vi "CorrelationTest2.vi"() -> ()   [LabVIEW 2014]
uses:
  <userlib>/Nanonis Prog Interface V5/Nanonis Prog Interface.lvlib
  <vilib>/Analysis/NI_AALPro.lvlib
  <vilib>/Analysis/2dsp.llb/2D Cross Correlation (DBL).vi
panel:
  out "Pixelated 2":picture
  out "Y drift 2":i32
  out "X drift 2":i32
  out "Pixelated":picture
  in  "length":i32
  in  "Boolean 2":bool
  in  "Filter order (2)":i32=2 min=1 max=1000 step=1
  in  "Cutoff frq (0.125)":dbl=0.125
  out "Array 2":dbl[][](array[numeric])
  out "min index(es)":i32[](array[numeric])
  in  "Numeric":i32
  out "shifted":picture
  out "Y drift":i32
  out "X drift":i32
  in  "method":i32 min=0 max=5
  in  "Boolean":bool
  out "Array":dbl[][](array[numeric])
  out "Rxy":dbl[][](array[numeric])
  out "max index(es)":i32[](array[numeric])=[127, 127]
  out "error":i32
  out "norm":picture
  out "no norm":picture
  in  "Read channel 2":i8 min=-1
  in  "algorithm":enum32{"direct", "frequency domain"}(ring)=enum."frequency domain"
  out "Correlation":picture
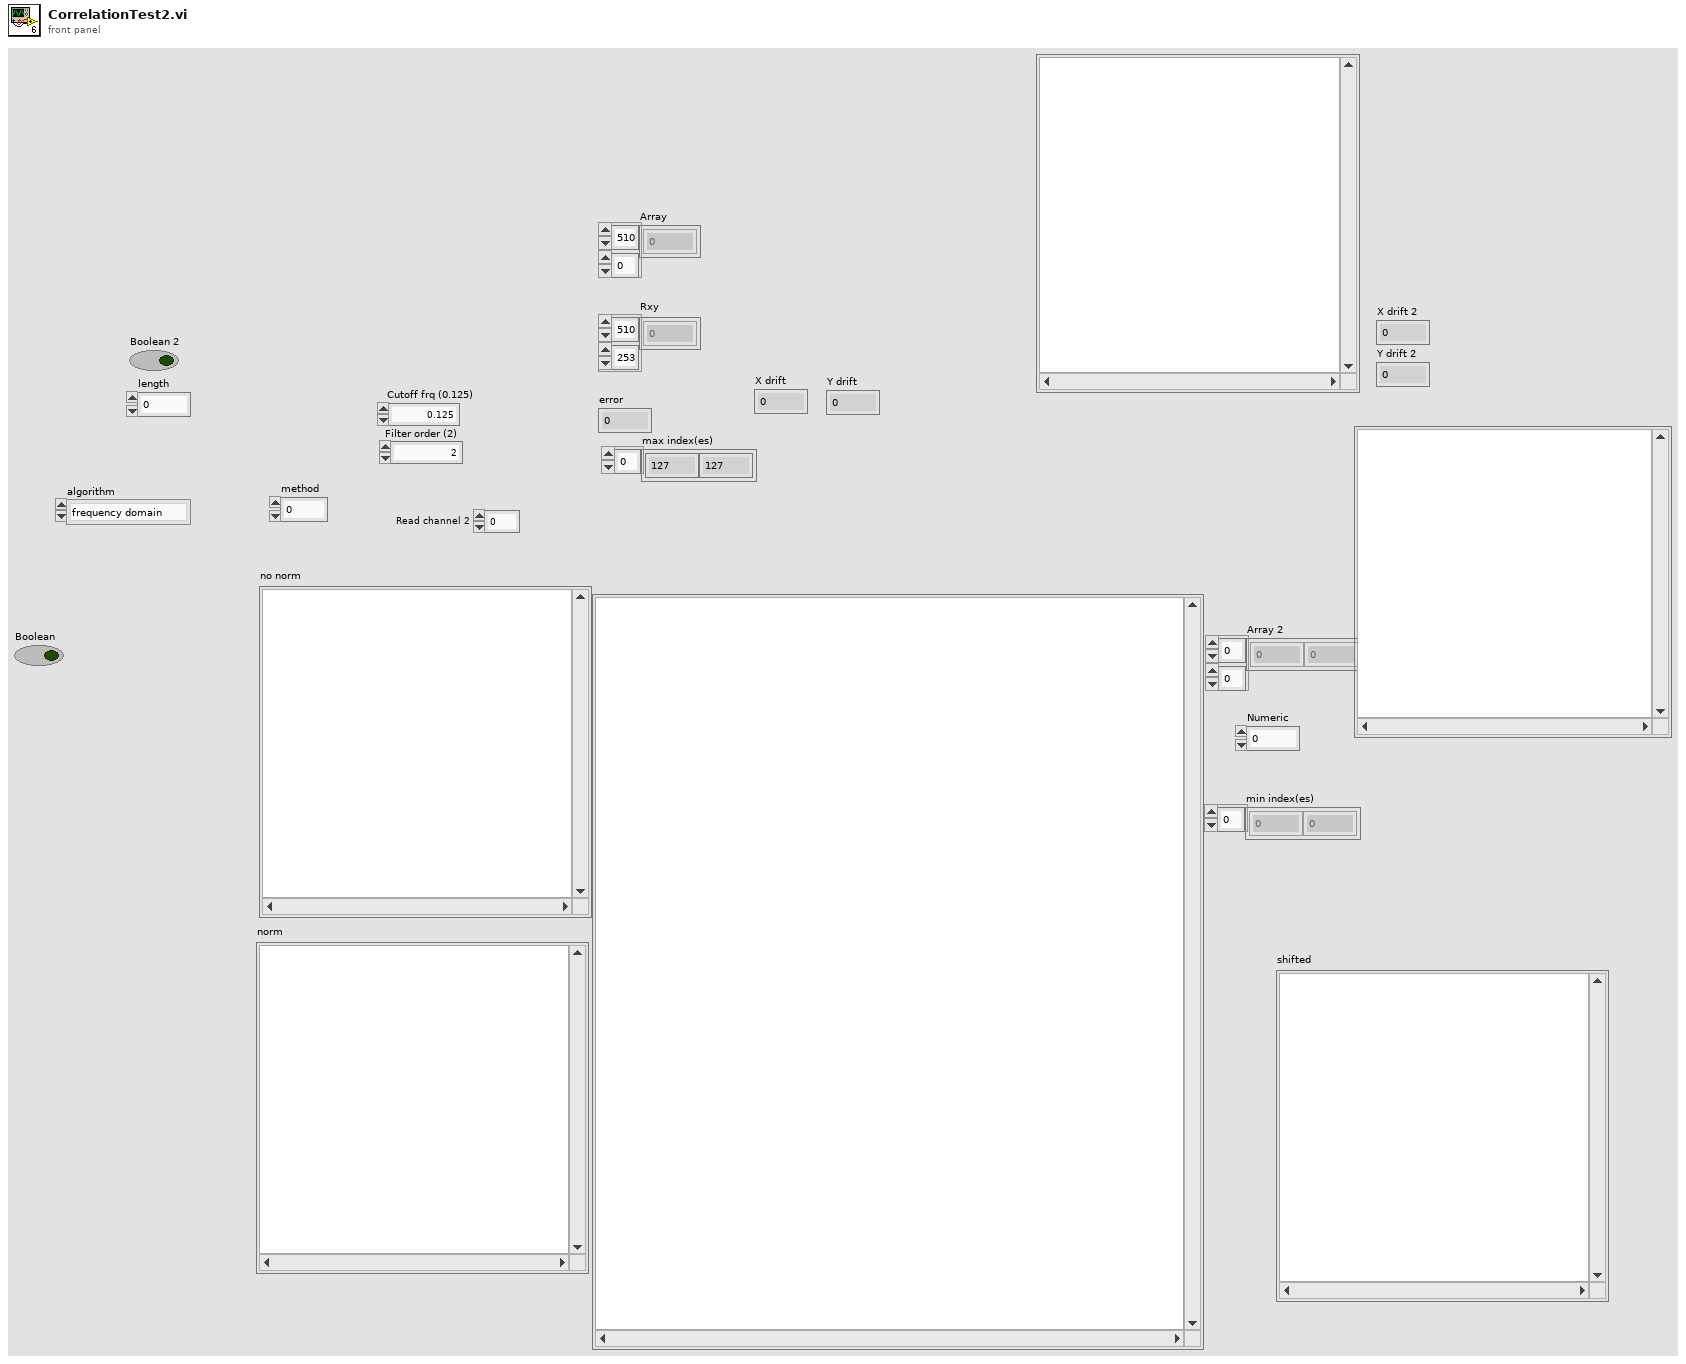
[diagram p1: front panel]
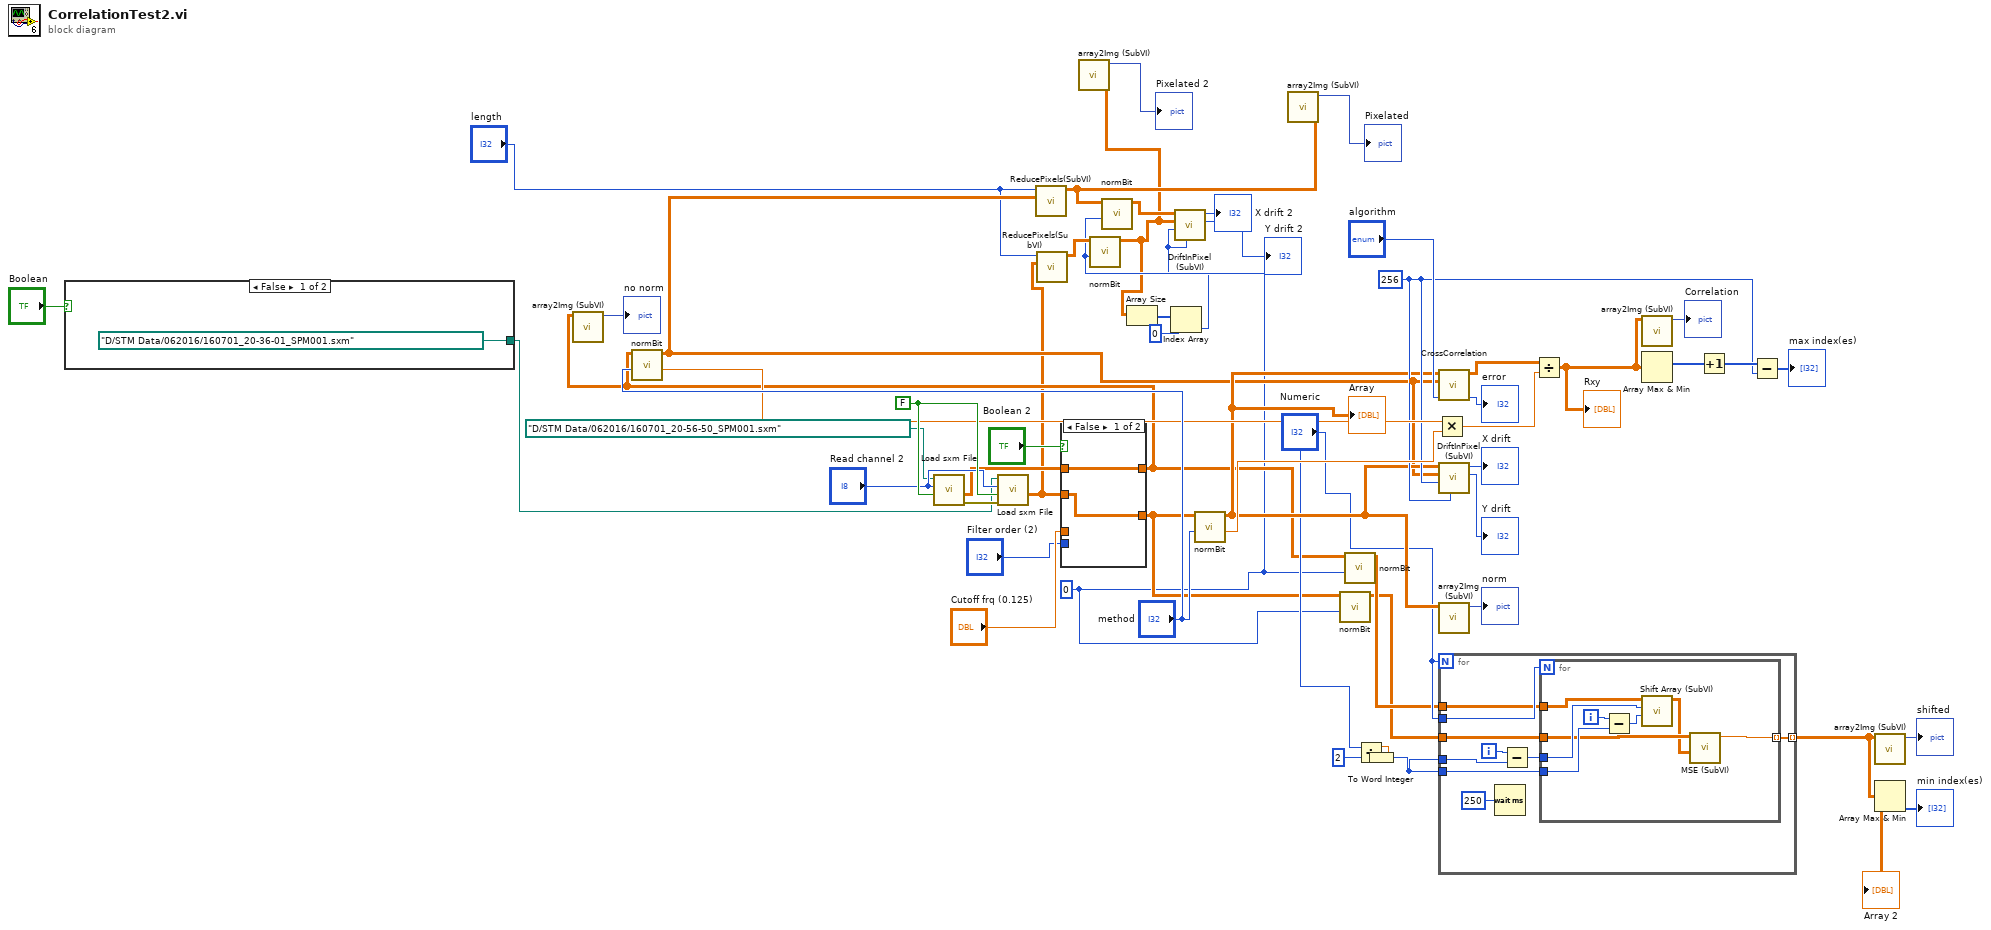
[diagram p0: block diagram]
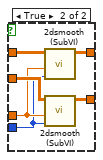
[diagram p2: hidden frame]
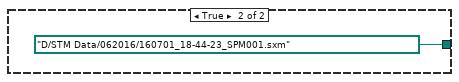
[diagram p3: hidden frame]
diagram:
  w6 = 0 ("method")
  w34 = 256
  w52 = FALSE ("Scan direction")
  n1 = case shown="False" "Boolean" {
    tunnel: [path "D:/STM Data/062016/160701_20-36-01_SPM001.sxm" ("Scan data file") path "D:/STM Data/062016/160701_18-44-23_SPM001.sxm" ("Scan data file")] -> w41
    frame False {
    }
    frame True {
    }
  }
  n2 = call <userlib>:"Load sxm File.vi"("Scan direction"=w52, "Read channel"="Read channel 2", "Scan data file"=path "D:/STM Data/062016/160701_20-56-50_SPM001.sxm") -> ("error out"=w51:errorcluster, "Data"=w20:sgl[][])  [unwired: 3 in, 4 out]
  n3 = call <userlib>:"Load sxm File.vi"("error in"=w51, "Scan direction"=w52, "Read channel"="Read channel 2", "Scan data file"=w41) -> ("Data"=w12:sgl[][])  [unwired: 2 in, 5 out]
  n4 = call "ReducePixels(SubVI).vi"("Array in"=w12, "length"="length") -> ("Array out"=w11:dbl[][])  [unwired: 9 in]
  n5 = case shown="False" "Boolean 2" {
    tunnel: [w57 w64] -> w21
    tunnel: w12 -> [w57 w63]
    tunnel: w20 -> [w58 w62]
    tunnel: [w58 w61] -> w19
    tunnel: "Cutoff frq (0.125)" -> [_ w60]
    tunnel: "Filter order (2)" -> [_ w59]
    frame False {
    }
    frame True {
      n6 = call "2dsmooth (SubVI).vi"("Filter order (2)"=w59, "Cutoff frq (0.125)"=w60, "Data"=w62) -> ("Y out"=w61:dbl[][])  [unwired: 8 in]
      n7 = call "2dsmooth (SubVI).vi"("Filter order (2)"=w59, "Cutoff frq (0.125)"=w60, "Data"=w63) -> ("Y out"=w64:dbl[][])  [unwired: 8 in]
    }
  }
  n8 = call "array2Img (SubVI).vi"("Rxy"=w19) -> ("new picture"=→"no norm":picture)  [unwired: 10 in]
  n9 = call "normBit.vi"("method"="method", "Rxy"=w19) -> ("standard deviation"=w37:dbl, "Array"=w15:dbl[][])  [unwired: 8 in]
  n10 = call "ReducePixels(SubVI).vi"("Array in"=w15, "length"="length") -> ("Array out"=w10:dbl[][])  [unwired: 9 in]
  n11 = call "normBit.vi"("method"=w6, "Rxy"=w11) -> ("Array"=w1:dbl[][])  [unwired: 8 in, 1 out]
  n12 = call "array2Img (SubVI).vi"("Rxy"=w1) -> ("new picture"=→"Pixelated 2":picture)  [unwired: 10 in]
  n13 = call "normBit.vi"("method"=w6, "Rxy"=w10) -> ("Array"=w9:dbl[][])  [unwired: 8 in, 1 out]
  n14 = Array Size(array=w1) -> (size(s)=w5:i32[])
  n15 = Index Array(array=w5, index=0) -> (element=w4:i32)
  n16 = call "DriftInPixel (SubVI).vi"(6:w4, 9:w4, "New image"=w1, "Ref image"=w9) -> ("Y drift"=→"Y drift 2":i32, "X drift"=→"X drift 2":i32)  [unwired: 5 in, 1 out]
  n17 = call "normBit.vi"("method"="method", "Rxy"=w21) -> ("standard deviation"=w36:dbl, "Array"=w30:dbl[][])  [unwired: 8 in]
  "Array" <- w30
  n18 = call "array2Img (SubVI).vi"("Rxy"=w10) -> ("new picture"=→"Pixelated":picture)  [unwired: 10 in]
  n19 = call "normBit.vi"("method"=w6, "Rxy"=w21) -> ("Array"=w22:dbl[][])  [unwired: 8 in, 1 out]
  n20 = call "normBit.vi"("method"=w6, "Rxy"=w19) -> ("Array"=w23:dbl[][])  [unwired: 8 in, 1 out]
  n21 = Divide(x="Numeric", y=2) -> (x/y=w27:dbl)
  n22 = To Word Integer(number=w27) -> (16bit integer=w24:i16)
  n23 = Multiply(x=w37, y=w36) -> (x*y=w35:dbl)
  n24 = call-poly <vilib>:"CrossCorrelation.vi"("algorithm"="algorithm", "Y"=w15, "X"=w30) -> ("error"=→"error":i32, "Rxy"=w46:dbl[][])  [unwired: 7 in]
  n25 = call "DriftInPixel (SubVI).vi"(6:w34, 9:w34, "New image"=w15, "Ref image"=w30) -> ("Y drift"=→"Y drift":i32, "X drift"=→"X drift":i32)  [unwired: 5 in, 1 out]
  n26 = call "array2Img (SubVI).vi"("Rxy"=w30) -> ("new picture"=→"norm":picture)  [unwired: 10 in]
  n27 = for {
    N: "Numeric" -> [_]
    tunnel: w22 -> [w73]
    tunnel: "Numeric" -> [w72]
    tunnel: w24 -> [w69]
    tunnel: w24 -> [w68]
    tunnel: w23 -> [w67]
    tunnel: [w66] -> w29 mode=indexing
    i -> [w70]
    n28 = Wait (ms)(milliseconds to wait=u32 250) -> ()  [unwired: 1 out]
    n29 = Subtract(x=w70, y=w69) -> (x-y=w71:i32)
    n30 = for {
      N: w72 -> [_]
      tunnel: w73 -> [w77]
      tunnel: w71 -> [w81]
      tunnel: w68 -> [w79]
      tunnel: w67 -> [w76]
      tunnel: [w75] -> w66 mode=indexing
      i -> [w80]
      n31 = Subtract(x=w80, y=w79) -> (x-y=w78:i32)
      n32 = call "Shift Array (SubVI).vi"("shift Y"=w78, "shift X+"=w81, "Array in"=w76) -> ("Array out"=w74:dbl[][])  [unwired: 8 in]
      n33 = call "MSE (SubVI).vi"("Img"=w74, "Ref"=w77) -> ("MSError"=w75:dbl)  [unwired: 9 in]
    }
  }
  "Array 2" <- w29
  n34 = Divide(x=w46, y=w35) -> (x/y=w38:dbl[][])
  "Rxy" <- w38
  n35 = call "array2Img (SubVI).vi"("Rxy"=w38) -> ("new picture"=→"Correlation":picture)  [unwired: 10 in]
  n36 = Array Max & Min(array=w38) -> (max index (indices)=w43:i32[])  [unwired: 3 out]
  n37 = Increment(x=w43) -> (x+1=w42:i32[])
  n38 = Subtract(x=w42, y=w34) -> (x-y=→"max index(es)":i32[])
  n39 = call "array2Img (SubVI).vi"("Rxy"=w29) -> ("new picture"=→"shifted":picture)  [unwired: 10 in]
  n40 = Array Max & Min(array=w29) -> (min index (indices)=→"min index(es)":i32[])  [unwired: 3 out]
